vi "SEK2020v1VI4IrAteATubulação.vi"(8 "Parâmetros":T1={"Azul Max EV3 Cor"=17, "Azul Min EV3 Cor"=0, "Verde Max EV3 Cor"=6, "Verde Min EV3 Cor"=0, "Vermelho Max Ev3 Cor"=0, "Vermelho Min EV3 Cor"=0, "Chão EV3 Cor"=0.0, "Branco Max EV3 Cor"=0.0, "Branco Min EV3 Cor"=0.0, "Preto Max EV3 Cor"=0.0, "Preto Min EV3 Cor"=0.0, "Distância Tubulação"=0.0, "Distância Frontal"=0.0, "Amarelo Max EV3 Cor"=0.0, "Amarelo Min EV3 Cor"=0.0, "Distância Lateral"=0.0, "90°"=0.0, "180°"=0.0, "Seguidor de Linha"=0.0}, 10 "NXT/EV3":T2) -> (2 "NXT/EV3 2":T2)   [LabVIEW 2016]
uses:
  <vilib>/NXT/Subs/LVHSConnector.ctl
  <vilib>/NXT/LegoClasses/BrickReference/BrickReference.lvclass
  <vilib>/NXT/Block Support/NXT_OutputPort.ctl
  <vilib>/NXT/Block Support/NXT_InputPort.ctl
  <vilib>/NXT/Dual Mode Library/Sensors/Touch_Pressed.vi
  <vilib>/NXT/NXTIO Xnodes/NXTIONodeSubVIs/NXTMoveMotors.vi
  <vilib>/NXT/NXTIO Xnodes/NXTIONodeSubVIs/NXTStopMotors.vi
  <vilib>/NXT/NXTIO Xnodes/AddressXNode/NXTIOAddress.xnode
  <vilib>/NXT/NXTIO Xnodes/NXTIOXNode/NXTIO.xnode
panel:
  # "Sensor EV3 Cor"
  # "Sensor Ultrassônico"
  # "Sensor Giroscópio"
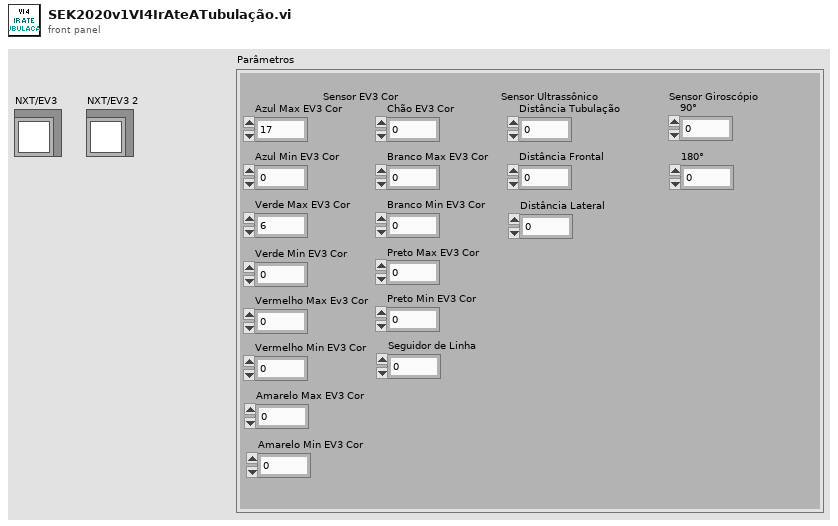
[diagram p1: front panel]
types:
  T1 = cluster{"Azul Max EV3 Cor":i32, "Azul Min EV3 Cor":i32, "Verde Max EV3 Cor":i32, "Verde Min EV3 Cor":i32, "Vermelho Max Ev3 Cor":i32, "Vermelho Min EV3 Cor":i32, "Chão EV3 Cor":sgl, "Branco Max EV3 Cor":sgl, "Branco Min EV3 Cor":sgl, "Preto Max EV3 Cor":sgl, "Preto Min EV3 Cor":sgl, "Distância Tubulação":sgl, "Distância Frontal":sgl, "Amarelo Max EV3 Cor":dbl, "Amarelo Min EV3 Cor":dbl, "Distância Lateral":sgl, "90°":sgl, "180°":sgl, "Seguidor de Linha":dbl}
  T2 = typedef "LVHSConnector.ctl" = refnum<class "BrickReference.lvclass">
  T3 = typedef "NXT_InputPort.ctl" = u32
  T4 = typedef "NXT_OutputPort.ctl" = u8
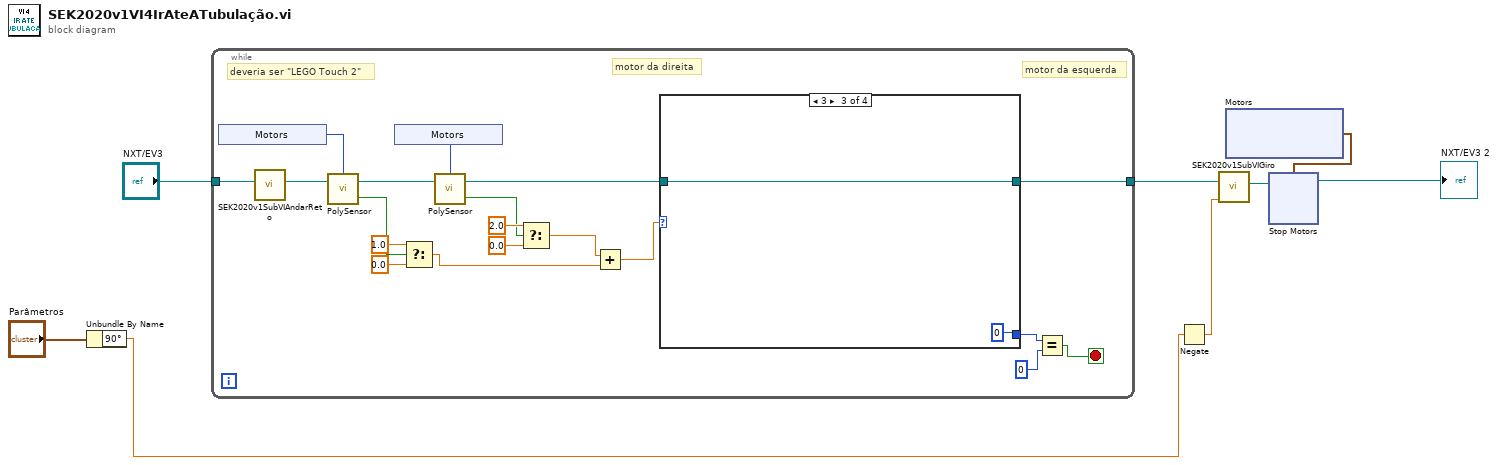
[diagram p0: block diagram]
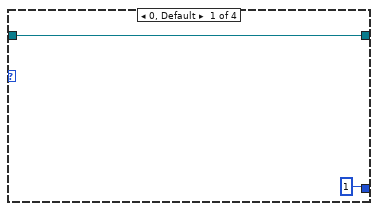
[diagram p2: hidden frame]
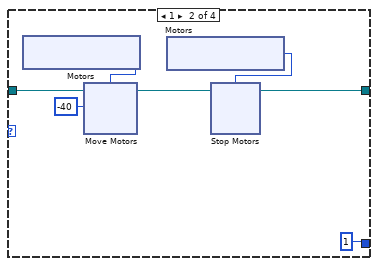
[diagram p3: hidden frame]
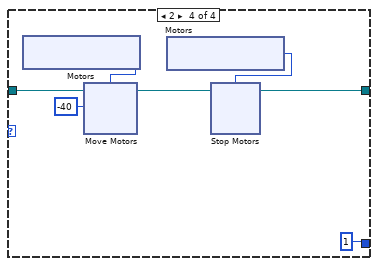
[diagram p4: hidden frame]
diagram:
  n1 = Unbundle By Name("Parâmetros") -> ("90°"=w2:sgl)
  n2 = while {
    tunnel: "NXT/EV3" -> [w22]
    tunnel: [w9] -> w6
    stop <- w24 stop-if-true
    # "motor da direita"
    # "motor da esquerda"
    # "deveria ser \"LEGO Touch 2\""
    n3 = xnode "Motors"() -> ("Sensor"=w26:T3)
    n4 = call "SEK2020v1SubVIAndarReto.vi"("NXT/EV3"=w22) -> ("NXT/EV3 2"=w21:T2)  [unwired: 9 in]
    n5 = call-poly <vilib>:"PolySensor.vi"("NXT/EV3"=w21, "Port (Port 1)"=w26) -> ("Yes / No"=w20:bool, "NXT/EV3"=w23:T2)  [unwired: 1 in]
    n6 = xnode "Motors"() -> ("Sensor"=w27:T3)
    n7 = Select(t=1.0, s=w20, f=0.0) -> (s? t:f=w12:dbl)
    n8 = call-poly <vilib>:"PolySensor.vi"("NXT/EV3"=w23, "Port (Port 1)"=w27) -> ("Yes / No"=w15:bool, "NXT/EV3"=w14:T2)  [unwired: 1 in]
    n9 = Select(t=2.0, s=w15, f=0.0) -> (s? t:f=w13:dbl)
    n10 = Add(x=w13, y=w12) -> (x+y=w11:dbl)
    n11 = case shown="3" w11 {
      tunnel: w14 -> [w29 w36 w52 w59]
      tunnel: [w29 w32 w52 w55] -> w9
      tunnel: [1 1 0 1] -> w10
      frame 0, Default {
      }
      frame 1 {
        n12 = xnode "Motors"() -> ("Motor"=w35:T4)
        n13 = xnode "Move Motors"("Power/Speed 1"=i8 -40, "Motors"=w35, "NXT/EV3"=w36) -> ("NXT/EV3"=w33:T2)
        n14 = xnode "Motors"() -> ("Motor"=w31:T4)
        n15 = xnode "Stop Motors"("Motors"=w31, "NXT/EV3"=w33) -> ("NXT/EV3"=w32:T2)
      }
      frame 3 {
      }
      frame 2 {
        n16 = xnode "Motors"() -> ("Motor"=w58:T4)
        n17 = xnode "Move Motors"("Power/Speed 1"=i8 -40, "Motors"=w58, "NXT/EV3"=w59) -> ("NXT/EV3"=w56:T2)
        n18 = xnode "Motors"() -> ("Motor"=w54:T4)
        n19 = xnode "Stop Motors"("Motors"=w54, "NXT/EV3"=w56) -> ("NXT/EV3"=w55:T2)
      }
    }
    n20 = Equal?(x=w10, y=0) -> (x = y?=w24:bool)
  }
  n21 = Negate(x=w2) -> (-x=w1:sgl)
  n22 = call "SEK2020v1SubVIGiro.vi"("ANGULO"=w1, "NXT/EV3"=w6) -> ("NXT/EV3 2"=w7:T2)  [unwired: 7 in]
  n23 = xnode "Motors"() -> ("Motor"=w4:cluster{"Port":T4, "Port":T4})
  n24 = xnode "Stop Motors"("Motors"=w4, "NXT/EV3"=w7) -> ("NXT/EV3"=→"NXT/EV3 2":T2)
